vi "Is Ball In Range.vi"(11 "Traj Pos Points in":cluster{"x":dbl, "y":dbl, "th":dbl}[](array[cluster])=[{"x"=18.101808459511187, "y"=17.986630843753836, "th"=0.0}, {"x"=18.098969470633545, "y"=17.994960318056133, "th"=-0.14400000000000002}, {"x"=18.093291492878258, "y"=18.011619266660727, "th"=-0.3766658248901368}, {"x"=18.08477452624533, "y"=18.036607689567617, "th"=-0.6093316497802735}, {"x"=18.073418570734756, "y"=18.069925586776804, "th"=-0.8419974746704103}, {"x"=18.05922362634654, "y"=18.11157295828829, "th"=-1.074663299560547}, {"x"=18.042189693080683, "y"=18.16154980410207, "th"=-1.3073291244506837}, {"x"=18.02231677093718, "y"=18.219856124218143, "th"=-1.5399949493408205}, {"x"=17.999604859916037, "y"=18.286491918636514, "th"=-1.7726607742309572}, {"x"=17.974053960017248, "y"=18.361457187357182, "th"=-2.005326599121094}, {"x"=17.945664071240817, "y"=18.444751930380146, "th"=-2.2379924240112303}, {"x"=17.91443519358674, "y"=18.536376147705408, "th"=-2.470658248901367}, {"x"=17.880367327055023, "y"=18.636329839332966, "th"=-2.7033240737915034}, {"x"=17.843460471645663, "y"=18.74461300526282, "th"=-2.93598989868164}, {"x"=17.80371462735866, "y"=18.861225645494972, "th"=-3.1686557235717765}, {"x"=17.761129794194012, "y"=18.98616776002942, "th"=-3.401321548461913}, {"x"=17.71596406204969, "y"=19.11868212392959, "th"=-3.6339873733520496}, {"x"=17.670798329905367, "y"=19.251196487829763, "th"=-3.866653198242186}, {"x"=17.625632597761044, "y"=19.383710851729933, "th"=-4.099319023132323}, {"x"=17.58046686561672, "y"=19.516225215630104, "th"=-4.33198484802246}, {"x"=17.535301133472398, "y"=19.648739579530275, "th"=-4.564650672912596}, {"x"=17.490135401328075, "y"=19.781253943430446, "th"=-4.797316497802733}, {"x"=17.444969669183752, "y"=19.913768307330617, "th"=-5.029982322692869}, {"x"=17.39980393703943, "y"=20.046282671230788, "th"=-5.262648147583006}, {"x"=17.354638204895107, "y"=20.17879703513096, "th"=-5.495313972473142}, {"x"=17.309472472750784, "y"=20.31131139903113, "th"=-5.727979797363279}, {"x"=17.26430674060646, "y"=20.4438257629313, "th"=-5.960645622253415}, {"x"=17.219141008462138, "y"=20.57634012683147, "th"=-6.193311447143552}, {"x"=17.173975276317815, "y"=20.708854490731643, "th"=-6.4259772720336885}, {"x"=17.128809544173492, "y"=20.841368854631813, "th"=-6.658643096923825}, {"x"=17.08364381202917, "y"=20.973883218531984, "th"=-6.891308921813962}, {"x"=17.038478079884847, "y"=21.106397582432155, "th"=-7.123974746704098}, {"x"=16.993312347740524, "y"=21.238911946332326, "th"=-7.356640571594235}, {"x"=16.9481466155962, "y"=21.371426310232497, "th"=-7.589306396484371}, {"x"=16.902980883451878, "y"=21.503940674132668, "th"=-7.821972221374508}, {"x"=16.857815151307555, "y"=21.63645503803284, "th"=-8.054638046264644}, {"x"=16.812649419163233, "y"=21.76896940193301, "th"=-8.287303871154782}, {"x"=16.76748368701891, "y"=21.90148376583318, "th"=-8.51996969604492}, {"x"=16.722317954874587, "y"=22.03399812973335, "th"=-8.752635520935057}, {"x"=16.677152222730264, "y"=22.166512493633522, "th"=-8.985301345825194}, {"x"=16.63198649058594, "y"=22.299026857533693, "th"=-9.217967170715331}, {"x"=16.58682075844162, "y"=22.431541221433864, "th"=-9.450632995605469}, {"x"=16.541655026297295, "y"=22.564055585334035, "th"=-9.683298820495606}, {"x"=16.496489294152973, "y"=22.696569949234206, "th"=-9.915964645385744}, {"x"=16.45132356200865, "y"=22.829084313134377, "th"=-10.148630470275881}, {"x"=16.406157829864327, "y"=22.961598677034548, "th"=-10.381296295166019}, {"x"=16.360992097720004, "y"=23.09411304093472, "th"=-10.613962120056156}, {"x"=16.31582636557568, "y"=23.22662740483489, "th"=-10.846627944946293}, {"x"=16.27066063343136, "y"=23.35914176873506, "th"=-11.07929376983643}, {"x"=16.225494901287036, "y"=23.49165613263523, "th"=-11.311959594726568}, {"x"=16.180329169142713, "y"=23.624170496535402, "th"=-11.544625419616706}, {"x"=16.13516343699839, "y"=23.756684860435573, "th"=-11.777291244506843}, {"x"=16.089997704854067, "y"=23.889199224335744, "th"=-12.00995706939698}, {"x"=16.044831972709744, "y"=24.021713588235915, "th"=-12.242622894287118}, {"x"=15.999666240565421, "y"=24.154227952136086, "th"=-12.475288719177255}, {"x"=15.954500508421098, "y"=24.286742316036257, "th"=-12.707954544067393}, {"x"=15.909334776276776, "y"=24.419256679936428, "th"=-12.94062036895753}, {"x"=15.864169044132453, "y"=24.5517710438366, "th"=-13.173286193847668}, {"x"=15.81900331198813, "y"=24.68428540773677, "th"=-13.405952018737805}, {"x"=15.773837579843807, "y"=24.81679977163694, "th"=-13.638617843627943}, {"x"=15.728671847699484, "y"=24.94931413553711, "th"=-13.87128366851808}, {"x"=15.683506115555161, "y"=25.081828499437282, "th"=-14.103949493408217}, {"x"=15.638340383410839, "y"=25.214342863337453, "th"=-14.336615318298355}, {"x"=15.593174651266516, "y"=25.346857227237624, "th"=-14.569281143188492}, {"x"=15.548008919122193, "y"=25.479371591137795, "th"=-14.80194696807863}, {"x"=15.50284318697787, "y"=25.611885955037966, "th"=-15.034612792968767}, {"x"=15.457677454833547, "y"=25.744400318938137, "th"=-15.267278617858905}, {"x"=15.412511722689224, "y"=25.876914682838308, "th"=-15.499944442749042}, {"x"=15.367345990544901, "y"=26.00942904673848, "th"=-15.73261026763918}, {"x"=15.322180258400579, "y"=26.14194341063865, "th"=-15.965276092529317}, {"x"=15.277014526256256, "y"=26.27445777453882, "th"=-16.197941917419453}, {"x"=15.231848794111933, "y"=26.40697213843899, "th"=-16.43060774230959}, {"x"=15.18668306196761, "y"=26.539486502339162, "th"=-16.663273567199727}, {"x"=15.141517329823287, "y"=26.672000866239333, "th"=-16.895939392089865}, {"x"=15.099190586556608, "y"=26.796185755837207, "th"=-17.128605216980002}, {"x"=15.059702832167572, "y"=26.91204117113279, "th"=-17.36127104187014}, {"x"=15.02305406665618, "y"=27.019567112126072, "th"=-17.593936866760277}, {"x"=14.989244290022429, "y"=27.11876357881706, "th"=-17.826602691650415}, {"x"=14.958273502266321, "y"=27.20963057120575, "th"=-18.059268516540552}, {"x"=14.930141703387857, "y"=27.292168089292144, "th"=-18.29193434143069}, {"x"=14.904848893387037, "y"=27.36637613307624, "th"=-18.524600166320827}, {"x"=14.88239507226386, "y"=27.43225470255804, "th"=-18.757265991210964}, {"x"=14.862780240018326, "y"=27.489803797737544, "th"=-18.9899318161011}, {"x"=14.846004396650434, "y"=27.53902341861475, "th"=-19.22259764099124}, {"x"=14.832067542160186, "y"=27.57991356518966, "th"=-19.455263465881377}, {"x"=14.82096967654758, "y"=27.612474237462273, "th"=-19.687929290771514}, {"x"=14.812710799812619, "y"=27.63670543543259, "th"=-19.798817024230978}, {"x"=14.8072909119553, "y"=27.652607159100608, "th"=-19.798817024230978}, {"x"=14.804710012975626, "y"=27.66017940846633, "th"=-19.8125}]) -> (3 "logical AND":bool=TRUE)   [LabVIEW 2025]
panel:
  in  "Rectangle Blue Alliance 2":T1(array[cluster])=[{"Left"=25, "Top"=422, "Right"=292, "Bottom"=317}, {"Left"=55, "Top"=444, "Right"=132, "Bottom"=422}, {"Left"=185, "Top"=444, "Right"=262, "Bottom"=422}]
  out "size(s) 2":i32=89
  out "size(s)":i32=89
  out "Image Out":T2(plugin-control)
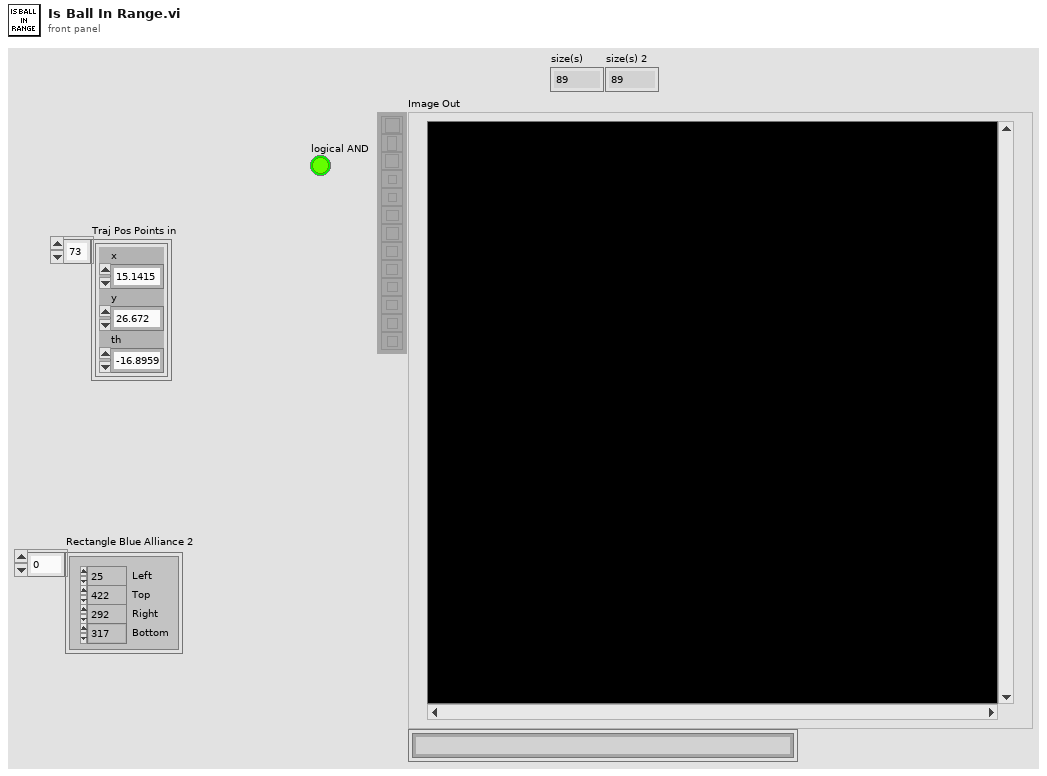
[diagram p1: front panel]
types:
  T1 = cluster{"Left":i32, "Top":i32, "Right":i32, "Bottom":i32}[]
  T2 = typedef "IMAQ Image.ctl" = refnum<image>
  T3 = typedef "Image Type" = u32
  T4 = typedef "WPI_DriverStationAllianceInfo.ctl" = enum16{"Red", "Blue", "Invalid"}
  T5 = cluster{"Left":i32, "Top":i32, "Right":i32, "Bottom":i32}
  T6 = cluster{"Left":dbl, "Top":dbl, "Right":dbl, "Bottom":dbl}
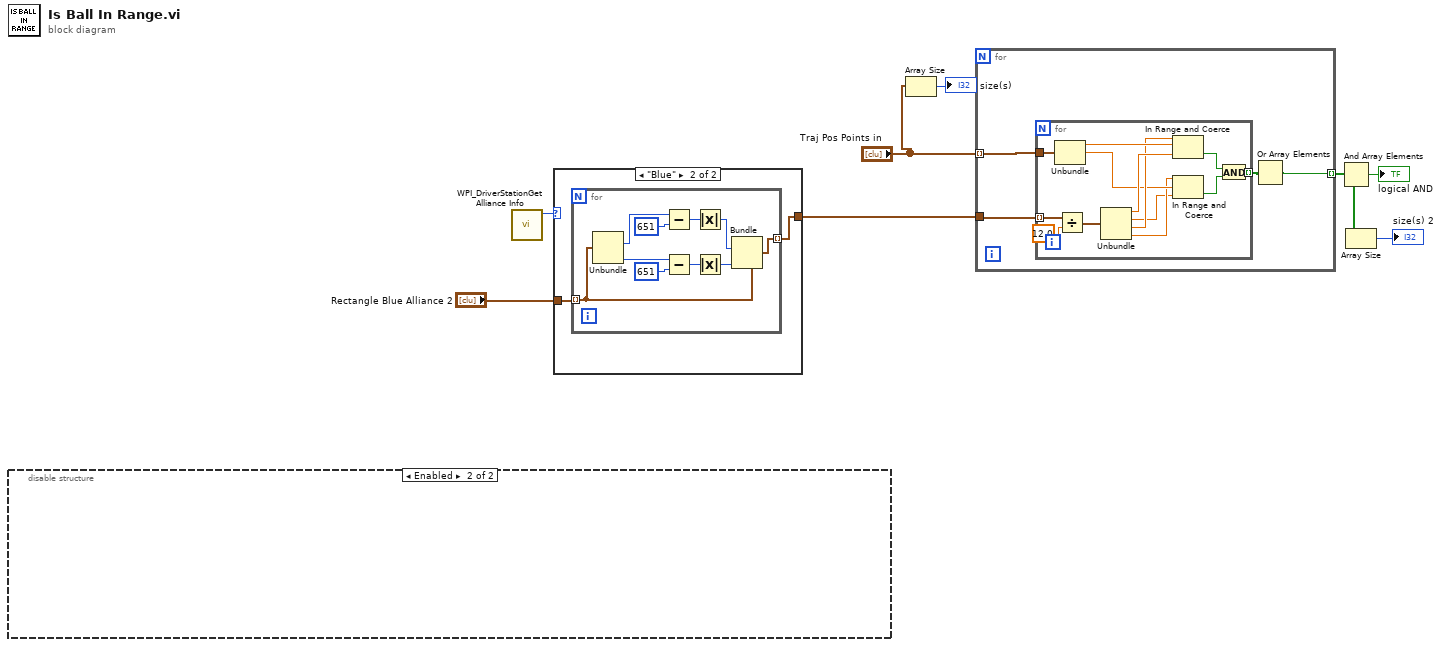
[diagram p0: block diagram]
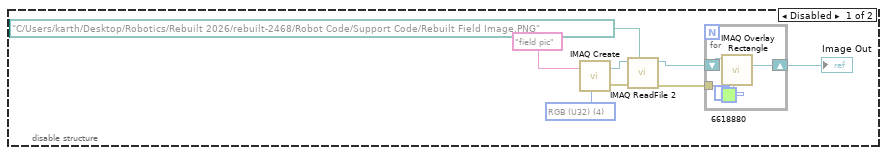
[diagram p3: hidden frame]
diagram:
  n1 = disable-structure shown="Enabled" {
    frame Disabled {
      w15 = T3 4 items=["Grayscale (U8)", "Grayscale (I16)", "Grayscale (SGL)", "Complex (CSG)", "RGB (U32)", "HSL (U32)", "RGB (U64)", "Grayscale (U16)"] ("Image Type")
      n2 = call "IMAQ Create"("Image Name"="field pic", "Image Type"=w15) -> ("New Image"=w13:T2, "error out"=w14:errorcluster)  [unwired: 3 in]
      n3 = call "IMAQ ReadFile 2"("File Path"=path "C:/Users/karth/Desktop/Robotics/Rebuilt 2026/rebuilt-2468/Robot Code/Support Code/Rebuilt Field Image.PNG", "error in (no error)"=w14, "Image"=w13) -> ("error out"=w11:errorcluster, "Image Out"=w10:T2)  [unwired: 4 in, 3 out]
      n4 = for {
        tunnel: w11 -> [w20]
        shift-right: [w18] -> w9
        shift-left: w10 -> [w19]
        n5 = call "IMAQ Overlay Rectangle"("Color"=u32 6618880, "error in (no error)"=w20, "Image"=w19) -> ("Image Out"=w18:T2)  [unwired: 7 in, 1 out]
      }
      "Image Out" <- w9
    }
    frame Enabled {
    }
  }
  n6 = call <vilib>:"WPI_DriverStationGet Alliance Info.vi"() -> ("Alliance"=w2:T4)  [unwired: 6 in, 5 out]
  n7 = case shown="\"Blue\"" w2 {
    tunnel: "Rectangle Blue Alliance 2" -> [w21 w23]
    tunnel: [w21 w22] -> w1
    frame "Red", Default {
    }
    frame "Blue" {
      n8 = for {
        tunnel: w23 -> [w28] mode=indexing
        tunnel: [w25] -> w22 mode=indexing
        n9 = Unbundle(w28) -> ("Top"=w33:i32, "Bottom"=w31:i32)  [unwired: 2 out]
        n10 = Subtract(x=w33, y=651) -> (x-y=w30:i32)
        n11 = Subtract(x=w31, y=651) -> (x-y=w29:i32)
        n12 = Absolute Value(x=w30) -> (abs(x)=w26:i32)
        n13 = Absolute Value(x=w29) -> (abs(x)=w27:i32)
        n14 = Bundle(cluster=w28, "Top"=w26, "Bottom"=w27) -> (w25:T5)  [unwired: 2 in]
      }
    }
  }
  n15 = Array Size(array="Traj Pos Points in") -> (size(s)=→"size(s)":i32)
  n16 = for {
    tunnel: "Traj Pos Points in" -> [w36] mode=indexing
    tunnel: w1 -> [w37]
    tunnel: [w34] -> w5 mode=indexing
    n17 = for {
      tunnel: w37 -> [w50] mode=indexing
      tunnel: w36 -> [w47]
      tunnel: [w40] -> w35 mode=indexing
      n18 = Unbundle(w47) -> ("x"=w46:dbl, "y"=w43:dbl)  [unwired: 1 out]
      n19 = Divide(x=w50, y=12.0) -> (x/y=w48:T6)
      n20 = Unbundle(w48) -> ("Left"=w45:dbl, "Top"=w38:dbl, "Right"=w44:dbl, "Bottom"=w39:dbl)
      n21 = In Range and Coerce(upper limit=w44, x=w46, lower limit=w45) -> (In Range?=w42:bool)  [unwired: 1 out]
      n22 = In Range and Coerce(upper limit=w39, x=w43, lower limit=w38) -> (In Range?=w41:bool)  [unwired: 1 out]
      n23 = And(x=w42, y=w41) -> (x .and. y?=w40:bool)
    }
    n24 = Or Array Elements(Boolean array=w35) -> (logical OR=w34:bool)
  }
  n25 = And Array Elements(Boolean array=w5) -> (logical AND=→"logical AND":bool)
  n26 = Array Size(array=w5) -> (size(s)=→"size(s) 2":i32)
